vi "open.vi"(8 "error in (no error)":errorcluster, 11 "IDeviceConnection in":refnum<class "IDeviceConnection.lvclass">) -> (0 "error out":errorcluster, 3 "IDeviceConnection out":refnum<class "IDeviceConnection.lvclass">)   [LabVIEW 2023, in "IDeviceConnection.lvclass"]
uses:
  IDeviceConnection.lvclass
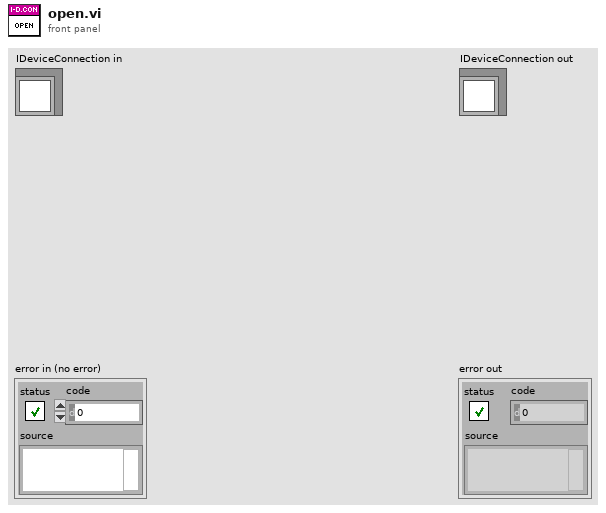
[diagram p1: front panel]
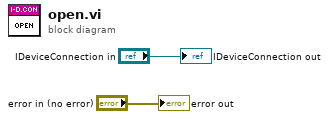
[diagram p0: block diagram]
diagram:
  "error out" <- "error in (no error)"
  "IDeviceConnection out" <- "IDeviceConnection in"
